vi "Data Analysis Test.vi"() -> ()   [LabVIEW 2021]
uses:
  Libraries/Data Analysis/Data Analysis.lvlib
panel:
  out "error out":errorcluster
  in  "Close Button":bool
  in  "View Button":bool
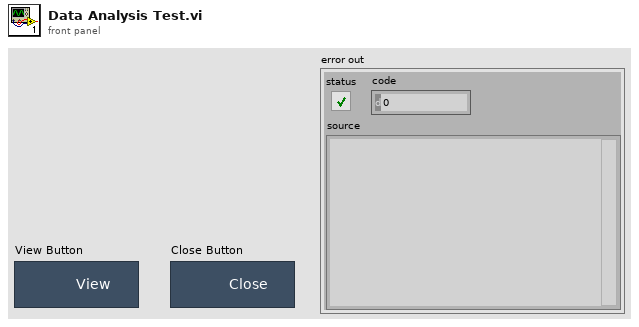
[diagram p1: front panel]
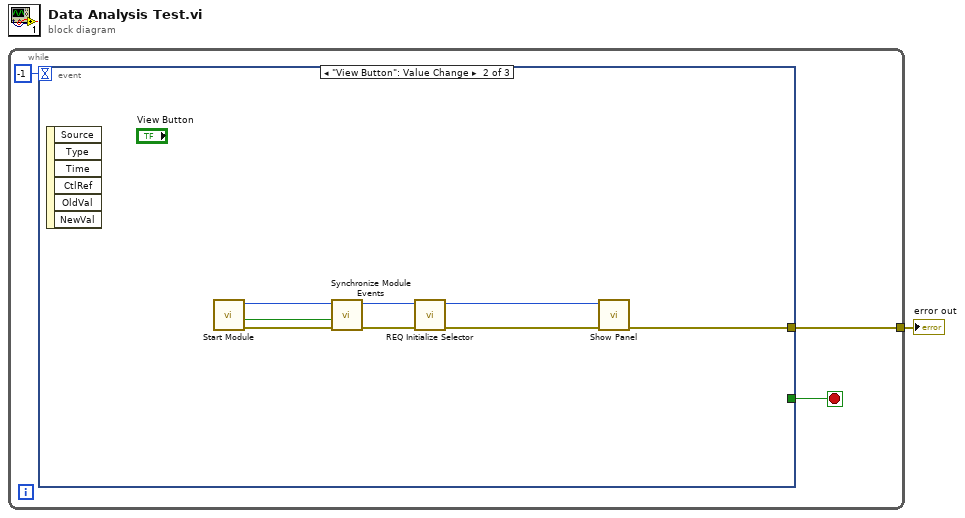
[diagram p0: block diagram]
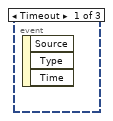
[diagram p2: hidden frame]
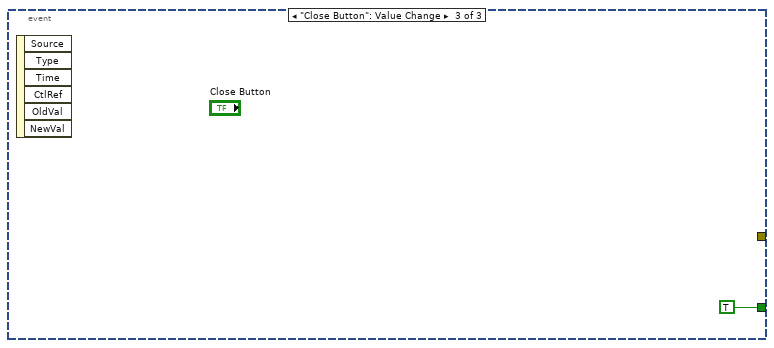
[diagram p3: hidden frame]
diagram:
  n1 = while {
    tunnel: [w2] -> w1
    stop <- w4 stop-if-true
    n2 = event shown="[1] \"View Button\": Value Change" {
      selector: _ -> [_ _ _]
      dyn-events: _ -> [_ _ _]
      timeout: -1 -> [_ _ _]
      tunnel: [_ _ TRUE] -> w4
      tunnel: [_ w5 _] -> w2
      event Timeout {
        n3 = event-data() -> ()  [unwired: 1 in, 3 out]
      }
      event "View Button": Value Change {
        n4 = event-data() -> ()  [unwired: 1 in, 6 out]
        n5 = call "Start Module.vi"() -> ("error out"=w11:errorcluster, "Wait for Event Sync?"=w10:bool, "Module ID"=w9:i32)  [unwired: 8 in, 1 out]
        n6 = call "Synchronize Module Events.vi"("error in"=w11, "Wait for Event Sync?"=w10, "Module ID in"=w9) -> ("error out"=w8:errorcluster, "Module ID out"=w6:i32)  [unwired: 7 in]
        n7 = call "REQ Initialize Selector.vi"("error in"=w8, "Module ID"=w6) -> ("error out"=w7:errorcluster)  [unwired: 9 in]
        n8 = call "Show Panel.vi"("error in (no error)"=w7, "Module ID"=w6) -> ("error out"=w5:errorcluster)  [unwired: 9 in]
      }
      event "Close Button": Value Change {
        n9 = event-data() -> ()  [unwired: 1 in, 6 out]
      }
    }
  }
  "error out" <- w1
